vi "PH_IEEE1394Camera.set Details to GUI.vi"(0 "VI in":refnum<vi>, 5 "error in (no error)":errorcluster) -> (14 "VI out":refnum<vi>, 19 "error out":errorcluster)   [LabVIEW 2014, in "PH_IEEE1394Camera.lvlib"]
uses:
  PH_IEEE1394Camera.lvlib
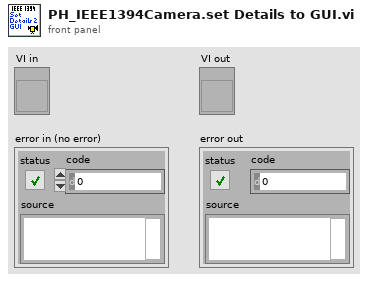
[diagram p1: front panel]
types:
  T1 = typedef "PH_IEEE1394Camera.lvlib/PH_IEEE1394Camera.i attribute.ctl" = cluster{"Gui Refs":cluster{"Brightness":refnum<vi>, "Shutter":refnum<vi>, "Gain":refnum<vi>, "Center of Gravity":refnum<vi>, "Supported Video Modes":refnum<vi>, "Trigger Polarity":refnum<vi>, "Trigger Mode":refnum<vi>, "Trigger Timeout":refnum<vi>, "Bit Depth":refnum<vi>, "Video Mode":refnum<vi>, "Top":refnum<vi>, "Bottom":refnum<vi>, "Left":refnum<vi>, "Right":refnum<vi>, "Set ROI to Maximum":refnum<vi>, "Camera Details":refnum<vi>, "Current Cam Attributes":refnum<vi>, "Attribute to set":refnum<vi>, "Num Value":refnum<vi>, "String Value":refnum<vi>, "Bool Value":refnum<vi>, "Set Cam Attribute":refnum<vi>}, "Cam":cluster{"IMAQ1394 Session":T2, "Camera Details":T3}, "Current Attributes":T4[], "Supported Video Modes ":cluster{"Video Mode":u32, "Video Mode Name":string}[], "Wanted Attributes":cluster{"Name":string, "Num Value":dbl, "String Value":string, "Boolean Value":bool}[], "Cam Attributes":T6}
  T2 = typedef "IMAQdx.ctl" = refnum<k21>
  T3 = typedef "PH_IEEE1394Camera.lvlib/PH_IEEE1394Camera.Cam Details.ctl" = cluster{"Model":string, "Serial Number":dbl, "Cam name (Machinery)":string, "Bus Type":string}
  T4 = typedef "PH_IEEE1394Camera.lvlib/PH_IEEE1394Camera.Cam Attribute.ctl" = cluster{"Information":cluster{"Type":T5, "Readable":bool, "Writable":bool, "Name":string}, "Num Value":dbl, "String Value":string, "Maximum":dbl, "Minimum":dbl, "Units":string, "Description":string, "EnumStrings[]":string[], "EnumValues[]":u32[], "Boolean Value":bool}
  T5 = typedef "NI_Vision_Acquisition_Software.lvlib/IMAQdx Attribute Type.ctl" = enum32{"U32", "I64", "DBL", "String", "Enum", "Bool", "Command"}
  T6 = typedef "PH_IEEE1394Camera.lvlib/PH_IEEE1394Camera.Relevant Cam Attributes.ctl" = cluster{"Video Mode":cluster{"Name":string, "Index":i32}, "Brightness":cluster{"Name":string, "Index":i32}, "Gain":cluster{"Name":string, "Index":i32}, "Shutter":cluster{"Name":string, "Index":i32}, "Trigger Pol":cluster{"Name":string, "Index":i32}, "Trigger Mode":cluster{"Name":string, "Index":i32}, "Timeout":cluster{"Name":string, "Index":i32}, "Bit Depth":cluster{"Name":string, "Index":i32}, "Pixel Bits":cluster{"Name":string, "Index":i32}, "Pixel Bytes":cluster{"Name":string, "Index":i32}, "Left":cluster{"Name":string, "Index":i32}, "Right":cluster{"Name":string, "Index":i32}, "Top":cluster{"Name":string, "Index":i32}, "Bottom":cluster{"Name":string, "Index":i32}}
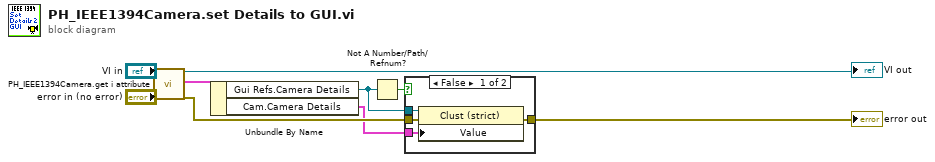
[diagram p0: block diagram]
diagram:
  n1 = call "PH_IEEE1394Camera.get i attribute.vi"("i ref in"="VI in", "error in (no error)"="error in (no error)") -> ("i ref out"=→"VI out":refnum<vi>, "i attribute"=w7:T1, "error out"=w8:errorcluster)  [unwired: 15 in]
  n2 = Unbundle By Name(w7) -> ("Gui Refs.Camera Details"=w5:refnum<vi>, "Cam.Camera Details"=w4:T3)
  n3 = Not A Number/Path/Refnum?(number/path/refnum=w5) -> (NaN/Path/Refnum?=w6:bool)
  n4 = case shown="False" w6 {
    tunnel: [w13 w14] -> w9
    tunnel: w8 -> [w12 w14]
    tunnel: w5 -> [w11 _]
    tunnel: w4 -> [w10 _]
    frame False {
      n5 = property class="Clust (strict)"(reference=w11, error in=w12, "Value"=w10) -> (error out=w13:errorcluster)  [unwired: 1 out]
    }
    frame True {
    }
  }
  "error out" <- w9
